vi "Add Frame Array File.vi"(7 "Highlight? (F)":bool, 8 "error in":errorcluster, 11 "Port Outgoing Ref":T1 format="%.0x") -> (0 "error out":errorcluster, 3 "Port Outgoing Ref out":T1 format="%.0x")   [LabVIEW 2020, in "AIM ARINC 664 Scripting.lvlib"]
uses:
  AIM ARINC 664 Scripting.lvlib
  <vilib>/NI VeriStand/Custom Device API/Custom Device Item Ref.ctl
  Constants.vi
  <vilib>/NI VeriStand/Custom Device API/Custom Device API.lvlib
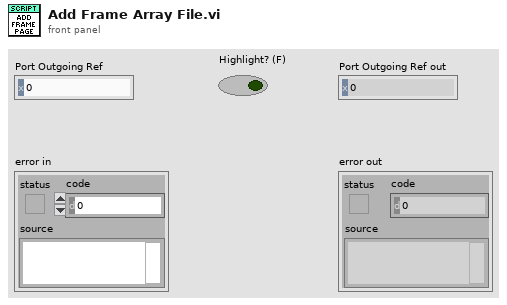
[diagram p1: front panel]
types:
  T1 = typedef "Custom Device API.lvlib/Custom Device Item Ref.ctl" = u64
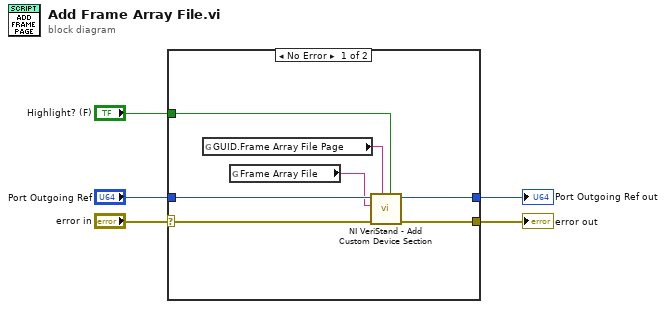
[diagram p0: block diagram]
diagram:
  n1 = case shown="No Error" "error in" {
    selector: "error in" -> [w9 w14]
    tunnel: "Highlight? (F)" -> [w11 _]
    tunnel: "Port Outgoing Ref" -> [w10 w13]
    tunnel: [w8 w14] -> w3
    tunnel: [w6 w13] -> w2
    frame No Error {
      n2 = global read "Constants.vi" "GUID.Frame Array File Page"() -> (w12:string)
      n3 = global read "Constants.vi" "Frame Array File"() -> (w7:string)
      n4 = call <vilib>:"NI VeriStand - Add Custom Device Section.vi"("Highlight? (F)"=w11, "GUID (Default Section)"=w12, "error in (no error)"=w9, "Section Name"=w7, "Parent Ref in"=w10) -> ("error out"=w8:errorcluster, "Parent Ref out"=w6:T1)  [unwired: 3 in, 2 out]
    }
    frame Error {
    }
  }
  "error out" <- w3
  "Port Outgoing Ref out" <- w2
